vi "PID2.vi"(6 "Rest_PI_theta":bool, 10 "input":dbl format="%.2f", 11 "setpoint":dbl format="%.2f") -> (3 "output":dbl)   [LabVIEW 2021]
uses:
  <vilib>/addons/control/pid/pid.llb/PID Advanced (DBL).vi
  <vilib>/addons/control/pid/NI_PID_pid.lvlib
panel:
  in  "output range":cluster{"output high":dbl, "output low":dbl}={"output high"=0.2, "output low"=-0.2} {"output low" format="%.2f"; "output high" format="%.2f"}
  in  "PID gains":T1={"proportional gain (Kc)"=0.4, "integral time (Ti, min)"=0.28, "derivative time (Td, min)"=0.0}
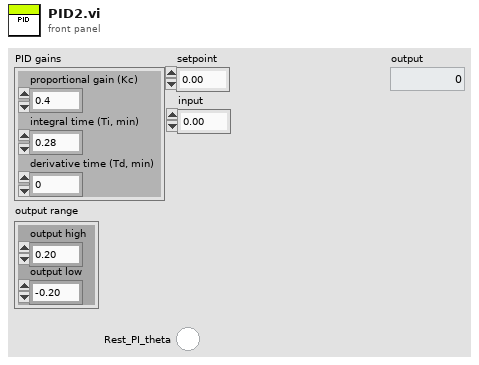
[diagram p1: front panel]
types:
  T1 = cluster{"proportional gain (Kc)":dbl, "integral time (Ti, min)":dbl, "derivative time (Td, min)":dbl}
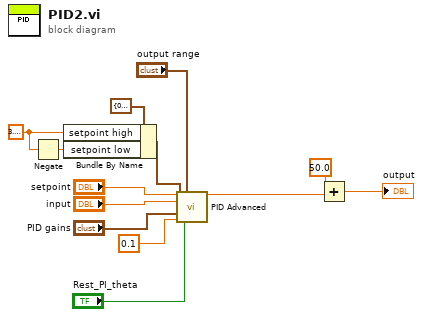
[diagram p0: block diagram]
diagram:
  w4 = 3.141592653589793
  n1 = Negate(x=w4) -> (-x=w3:dbl)
  n2 = Bundle By Name(cluster=cluster{"setpoint high":dbl, "setpoint low":dbl} {"setpoint high"=0.0, "setpoint low"=0.0} ("setpoint range"), "setpoint high"=w4, "setpoint low"=w3) -> (w6:cluster{"setpoint high":dbl, "setpoint low":dbl})
  n3 = call-poly <vilib>:"PID Advanced.vi"("setpoint"="setpoint", "output range"="output range", "process variable"="input", "setpoint range"=w6, "PID gains"="PID gains", "dt (s)"=0.1, "reinitialize? (F)"="Rest_PI_theta") -> ("output"=w10:dbl)  [unwired: 7 in, 1 out]
  n4 = Add(x=50.0, y=w10) -> (x+y=→"output":dbl)
